vi "SaveData.vi"(10 "DataFilePath":path, 11 "Products":T1[](array[typedef])) -> ()   [LabVIEW 2019]
uses:
  ProductsCluster.ctl
  <vilib>/Utility/file.llb/Write Delimited Spreadsheet (string).vi
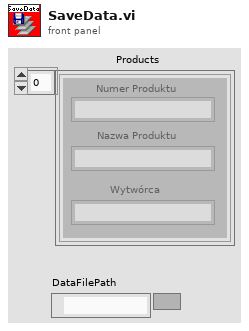
[diagram p1: front panel]
types:
  T1 = typedef "ProductsCluster.ctl" = cluster{"Numer Produktu":string, "Nazwa Produktu":string, "Wytwórca":string}
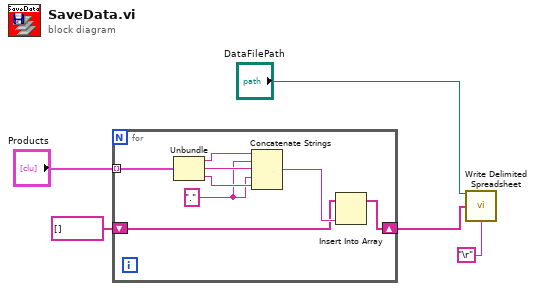
[diagram p0: block diagram]
diagram:
  n1 = for {
    shift-right: [w8] -> w2
    shift-left: string[] [] -> [w6]
    tunnel: "Products" -> [w13] mode=indexing
    w9 = "."
    n2 = Unbundle(w13) -> ("Numer Produktu"=w12:string, "Nazwa Produktu"=w11:string, "Wytwórca"=w10:string)
    n3 = Concatenate Strings(w12, w9, w11, w9, w10) -> (w7:string)
    n4 = Insert Into Array(array=w6, new element=w7) -> (w8:string[])  [unwired: 1 in]
  }
  n5 = call-poly <vilib>:"Write Delimited Spreadsheet.vi"("file path (dialog if empty)"="DataFilePath", "1D data"=w2, "delimiter (\\t)"="\r") -> ()  [unwired: 11 in, 2 out]
